vi "OKorCancel (Popup).vi"(0 "message":string, 1 "Seconds before TimeOut":dbl=200.0, 7 "T button name (\"OK\")":string, 9 "F button name (\"Cancel\")":string, 11 "error in (no error)":errorcluster) -> (4 "T button?":bool, 10 "Time Out?":bool, 15 "error out":errorcluster)   [LabVIEW 2012]
panel:
  out "x-y":dbl
  out "current time 2":timestamp
  out "current time":timestamp
  in  "Cancel":bool
  in  "OK":bool
  out "?":string
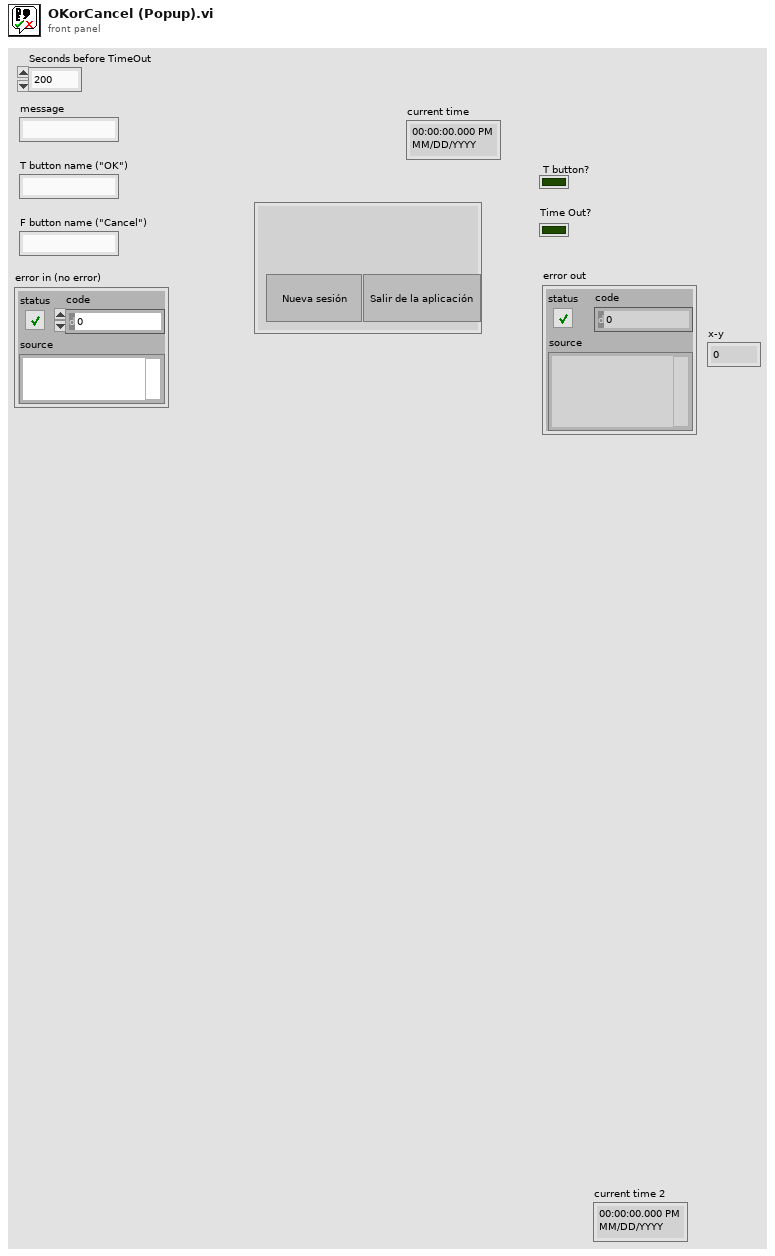
[diagram p1: front panel]
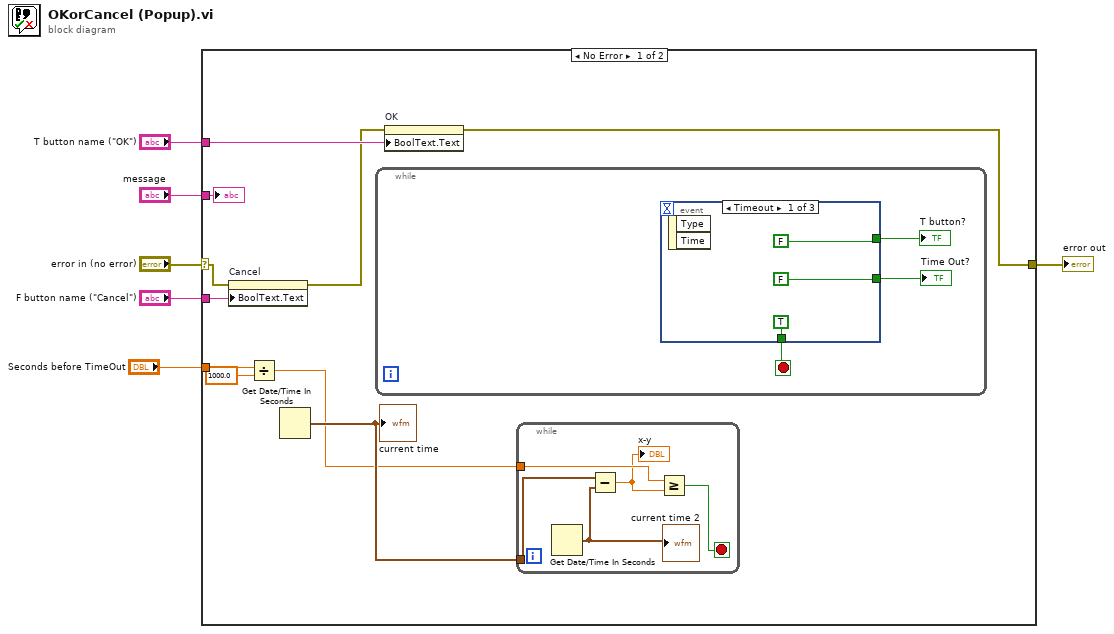
[diagram p0: block diagram]
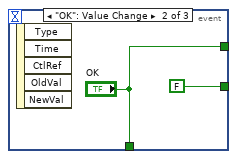
[diagram p2: hidden frame]
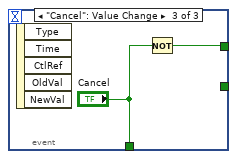
[diagram p3: hidden frame]
diagram:
  n1 = case shown="No Error" "error in (no error)" {
    selector: "error in (no error)" -> [w11 w32]
    tunnel: "T button name (\"OK\")" -> [w16 _]
    tunnel: [w15 w32] -> w5
    tunnel: "F button name (\"Cancel\")" -> [w14 _]
    tunnel: "message" -> [w12 _]
    tunnel: "Seconds before TimeOut" -> [w10 _]
    frame No Error {
      n2 = property on="Cancel" class="Bool"(error in=w11, "BoolText.Text"=w14) -> (error out=w13:errorcluster)  [unwired: 1 in, 1 out]
      n3 = Divide(x=w10, y=1000.0) -> (x/y=w7:dbl)
      n4 = Get Date/Time In Seconds() -> (seconds since 1Jan1904=w8:timestamp)
      "current time" <- w8
      n5 = while {
        stop <- w22 stop-if-true
        n6 = event shown="[0] Timeout" {
          selector: _ -> [_ _ _]
          dyn-events: _ -> [_ _ _]
          timeout: _ -> [_ _ _]
          tunnel: [FALSE FALSE _] -> w24
          tunnel: [FALSE "OK" w31] -> w23
          tunnel: [TRUE ("Cancel") "OK" "Cancel"] -> w22
          event Timeout {
            n7 = event-data() -> ()  [unwired: 1 in, 2 out]
          }
          event "OK": Value Change {
            n8 = event-data() -> ()  [unwired: 1 in, 5 out]
          }
          event "Cancel": Value Change {
            n9 = event-data() -> ()  [unwired: 1 in, 5 out]
            n10 = Not(x="Cancel") -> (.not. x?=w31:bool)
          }
        }
        "T button?" <- w23
        "Time Out?" <- w24
      }
      n11 = property on="OK" class="Bool"(error in=w13, "BoolText.Text"=w16) -> (error out=w15:errorcluster)  [unwired: 1 in, 1 out]
      n12 = while {
        tunnel: w8 -> [w21]
        tunnel: w7 -> [w19]
        stop <- w17 stop-if-true
        n13 = Get Date/Time In Seconds() -> (seconds since 1Jan1904=w20:timestamp)
        "current time 2" <- w20
        n14 = Subtract(x=w21, y=w20) -> (x-y=w18:dbl)
        "x-y" <- w18
        n15 = Greater Or Equal?(x=w19, y=w18) -> (x >= y?=w17:bool)
      }
      "?" <- w12
    }
    frame Error {
    }
  }
  "error out" <- w5
